vi "remote time.vi"(8 "Error In":errorcluster, 11 "server":string="bandicoot") -> (0 "Error Out":errorcluster, 1 "Local remote time":timestamp, 2 "Current time":timestamp, 3 "standard output":string)   [LabVIEW 2014]
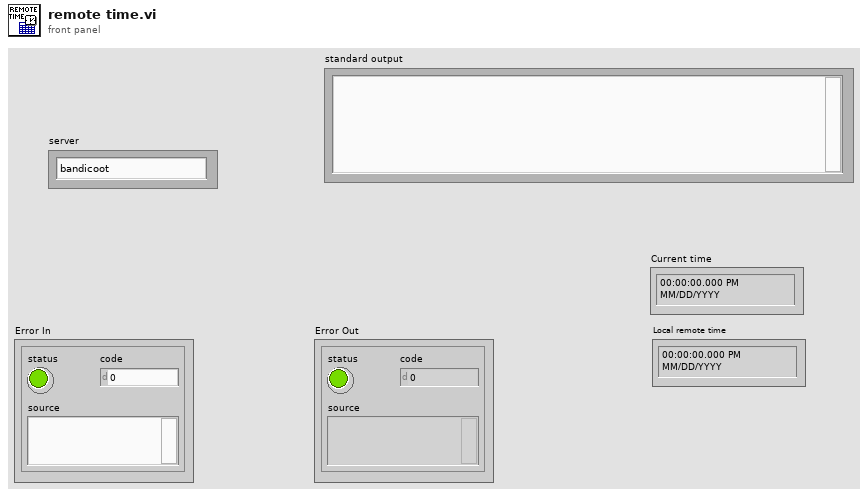
[diagram p1: front panel]
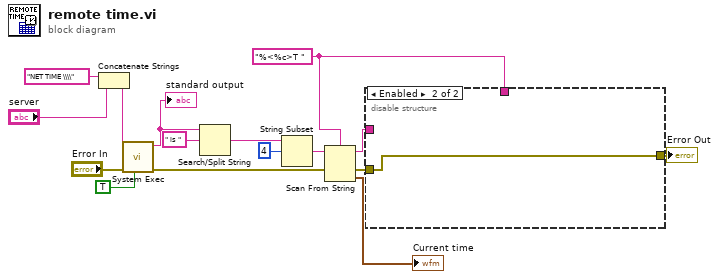
[diagram p0: block diagram]
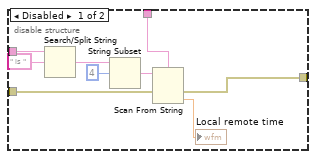
[diagram p2: hidden frame]
diagram:
  w8 = "%<%c>T " ("format string")
  n1 = Concatenate Strings("NET TIME \\\\" ("string"), "server") -> (w2:string)
  n2 = call <vilib>:"System Exec.vi"("run minimized? (F)"=TRUE, "error in (no error)"="Error In", "command line"=w2) -> ("error out"=w5:errorcluster, "standard output"=w14:string)  [unwired: 5 in, 2 out]
  "standard output" <- w14
  n3 = Search/Split String(string=w14, search string/char (-)=" is ") -> (match + rest of string=w12:string)  [unwired: 1 in, 2 out]
  n4 = String Subset(string=w12, offset (0)=4) -> (substring=w10:string)  [unwired: 1 in]
  n5 = Scan From String(format string=w8, input string=w10, error in=w5) -> (remaining string=w9:string, error out=w4:errorcluster, output 1=→"Current time":timestamp)  [unwired: 2 in, 1 out]
  n6 = disable-structure shown="Enabled" {
    disable-tunnel: w9 -> [w22 _]
    disable-tunnel: w8 -> [w20 _]
    disable-tunnel: w4 -> [w18 w26]
    disable-tunnel: [w17 w26] -> w3
    frame Disabled {
      n7 = Search/Split String(string=w22, search string/char (-)=" is ") -> (match + rest of string=w23:string)  [unwired: 1 in, 2 out]
      n8 = String Subset(string=w23, offset (0)=4) -> (substring=w21:string)  [unwired: 1 in]
      n9 = Scan From String(format string=w20, input string=w21, error in=w18) -> (error out=w17:errorcluster, output 1=→"Local remote time":dbl)  [unwired: 2 in, 2 out]
    }
    frame Enabled {
    }
  }
  "Error Out" <- w3
